vi "Driver_Logic.vi"(3 "Driving Style":u16(knob) scale=0.0..2.0) -> (0 "Brake_Out":dbl, 1 "Throttle_Out":dbl)   [LabVIEW 2025]
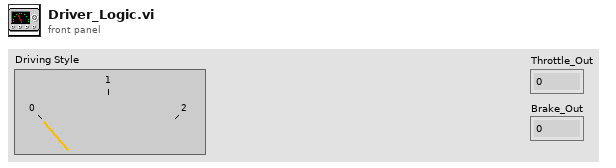
[diagram p1: front panel]
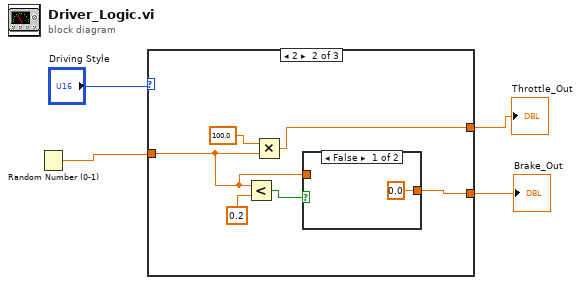
[diagram p0: block diagram]
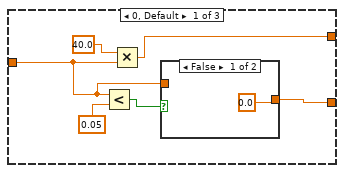
[diagram p2: hidden frame]
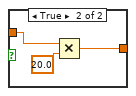
[diagram p3: hidden frame]
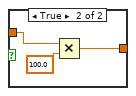
[diagram p4: hidden frame]
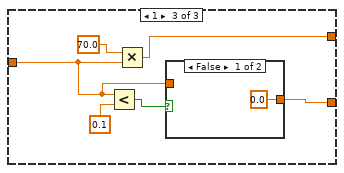
[diagram p5: hidden frame]
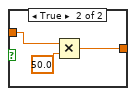
[diagram p6: hidden frame]
diagram:
  n1 = Random Number (0-1)() -> (number: 0 to 1=w3:dbl)
  n2 = case shown="2" "Driving Style" {
    tunnel: w3 -> [w7 w17 w27]
    tunnel: [w6 w15 w25] -> w1
    tunnel: [w5 w16 w26] -> w2
    frame 0, Default {
      n3 = Less?(x=w7, y=0.05) -> (x < y?=w8:bool)
      n4 = Multiply(x=40.0, y=w7) -> (x*y=w5:dbl)
      n5 = case shown="False" w8 {
        tunnel: w7 -> [_ w14]
        tunnel: [0.0 w12] -> w6
        frame False {
        }
        frame True {
          n6 = Multiply(x=w14, y=20.0) -> (x*y=w12:dbl)
        }
      }
    }
    frame 2 {
      n7 = Less?(x=w17, y=0.2) -> (x < y?=w18:bool)
      n8 = Multiply(x=100.0, y=w17) -> (x*y=w16:dbl)
      n9 = case shown="False" w18 {
        tunnel: w17 -> [_ w24]
        tunnel: [0.0 w22] -> w15
        frame False {
        }
        frame True {
          n10 = Multiply(x=w24, y=100.0) -> (x*y=w22:dbl)
        }
      }
    }
    frame 1 {
      n11 = Less?(x=w27, y=0.1) -> (x < y?=w28:bool)
      n12 = Multiply(x=70.0, y=w27) -> (x*y=w26:dbl)
      n13 = case shown="False" w28 {
        tunnel: w27 -> [_ w34]
        tunnel: [0.0 w32] -> w25
        frame False {
        }
        frame True {
          n14 = Multiply(x=w34, y=50.0) -> (x*y=w32:dbl)
        }
      }
    }
  }
  "Throttle_Out" <- w2
  "Brake_Out" <- w1
